vi "Search And Remove ID Priv.vi"(4 "Unique ID":string, 5 "Child IDs In":string[](array[string])) -> (2 "Child IDs Out":string[](array[string]))   [LabVIEW 2016, in "Tree Manager.lvclass"]
uses:
  Tree Manager.lvclass
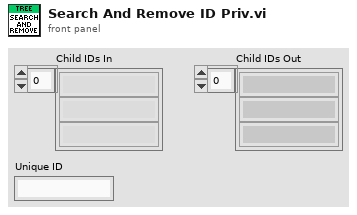
[diagram p1: front panel]
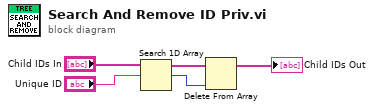
[diagram p0: block diagram]
diagram:
  n1 = Search 1D Array(1D array="Child IDs In", element="Unique ID") -> (index of element=w2:i32)  [unwired: 1 in]
  n2 = Delete From Array(array="Child IDs In", index=w2) -> (array with subset deleted=→"Child IDs Out":string[])  [unwired: 1 in, 1 out]
